vi "showDialog.vi"(0 "HB_Dialog in":refnum<class "HB_Dialog.lvclass">=refnum, 11 "error in (no error)":errorcluster) -> (4 "HB_Dialog out":refnum<class "HB_Dialog.lvclass">, 8 "Button Index":i16, 15 "error out":errorcluster)   [LabVIEW 2009, in "HB_Inherance_Example.lvlib" / "HB_Dialog.lvclass"]
doc: "Dynamic dispatch VI. Sub classes must implement the display of the dialog."
uses:
  HB_Dialog.lvclass
  HB_TwoButtonDiolog/HB_TwoButtonDiolog.lvclass
  lib.lib/HGF_LVC/HGF_Auxiliary/Severity.ctl
  lib.lib/HGF_LVC/HGF_Auxiliary/ErrorCode.ctl
  lib.lib/HGF_LVC/HGF_Auxiliary/HGF_Auxiliary.lvlib
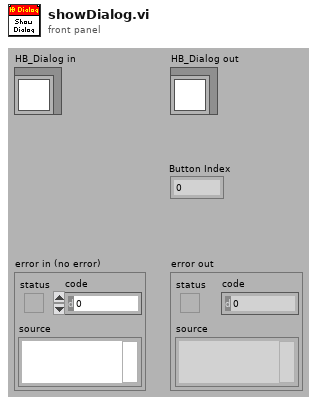
[diagram p1: front panel]
types:
  T1 = typedef "HGF_Auxiliary.lvlib/Severity.ctl" = enum16{"Info", "Warning", "Fault", "Error", "Fatal"}
  T2 = typedef "HGF_Auxiliary.lvlib/ErrorCode.ctl" = enum32{"No error", "Function not supported.", "This VI is for friends only.", "Reference object aready exisits.", "Parameter out of range.", "Not a rendezvous.", "Invalid notifier reference.", "Invalid queue reference.", "Self-Test not supported.", "Reset not supported.", "IDN query not supported.", "Error query not supported.", "Incorrect addressee.", "Object already exists.", "No class name specified", "Driver not supported", "Attribute is not writable"}
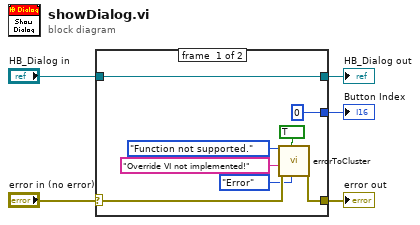
[diagram p0: block diagram]
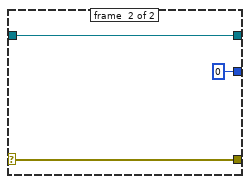
[diagram p2: hidden frame]
diagram:
  n1 = case shown="No Error" "error in (no error)" {
    selector: "error in (no error)" -> [w10 w16]
    tunnel: [w9 w16] -> w4
    tunnel: [w13 w15] -> w2
    tunnel: "HB_Dialog in" -> [w13 w15]
    tunnel: [i16 0 ("Button Index") i16 0 ("Button Index")] -> w1
    frame #0 {
      n2 = call "errorToCluster.vi"("error code"=ErrorCode."Function not supported.", "error message (\"\")"="Override VI not implemented!" ("error message (\"\")"), "error in (no error)"=w10, "show call chain? (True)"=TRUE, "severity (Error)"=Severity."Error") -> ("error out"=w9:errorcluster)  [unwired: 14 in]
    }
    frame #1 {
    }
  }
  "error out" <- w4
  "HB_Dialog out" <- w2
  "Button Index" <- w1
